vi "异步调用.vi"() -> ()   [LabVIEW 2011]
panel:
  in  "Stop Button":bool
  in  "Play Button":bool
  out "Gauge":dbl(knob) scale=0.0..10.0
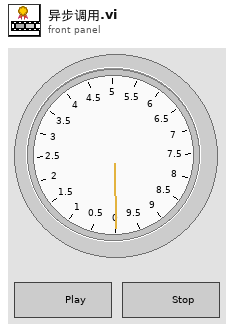
[diagram p1: front panel]
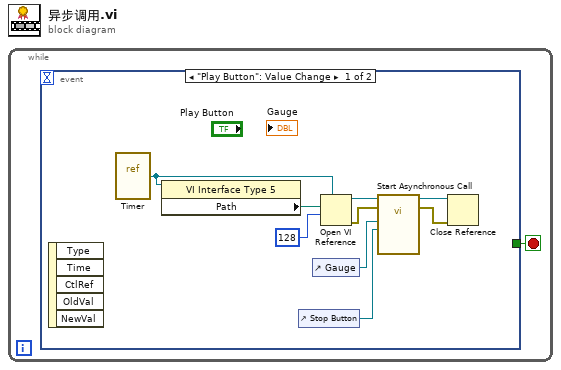
[diagram p0: block diagram]
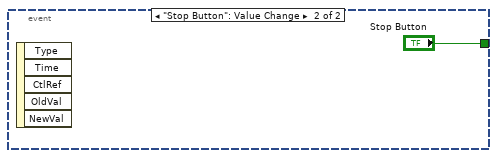
[diagram p2: hidden frame]
diagram:
  n1 = while {
    stop <- w1 stop-if-true
    n2 = event shown="[0] \"Play Button\": Value Change" {
      selector: _ -> [_ _]
      dyn-events: _ -> [_ _]
      timeout: _ -> [_ _]
      tunnel: [_ "Stop Button"] -> w1
      event "Play Button": Value Change {
        n3 = event-data() -> ()  [unwired: 1 in, 5 out]
        n4 = vi-ref "Timer.vi"() -> (w10:refnum<vi>)
        n5 = property class="VI Interface Type 5"(reference=w10) -> ("Path"=w9:path)  [unwired: 1 in, 2 out]
        n6 = control-ref of="Stop Button"() -> (w2:refnum<vi>)
        n7 = control-ref of="Gauge"() -> (w6:refnum<vi>)
        n8 = Open VI Reference(type specifier VI Refnum (for type only)=w10, vi path=w9, options=128) -> (vi reference=w7:refnum<vi>, error out=w5:errorcluster)  [unwired: 3 in]
        n9 = call-by-ref "Start Asynchronous Call"(reference=w7, error in=w5, "Stop Button"=w2, "Gauge"=w6) -> (reference out=w4:refnum<vi>, error out=w3:errorcluster)  [unwired: 10 in]
        n10 = Close Reference(reference=w4, error in (no error)=w3) -> ()  [unwired: 1 out]
      }
      event "Stop Button": Value Change {
        n11 = event-data() -> ()  [unwired: 1 in, 5 out]
      }
    }
  }
